vi "SR_Graph_compil_net_param (SubVI).vi"(4 "String":string, 6 "Int32":i32, 7 "String 4":string, 8 "Boolean":bool, 10 "String 2":string, 11 "Boolean 2":bool) -> (3 "String 3":string)   [LabVIEW 2018]
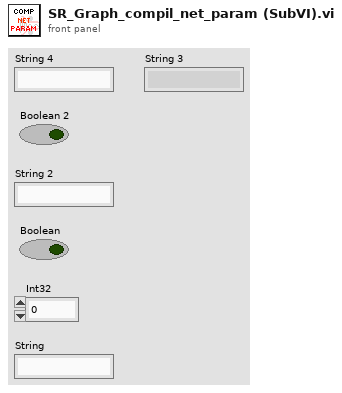
[diagram p1: front panel]
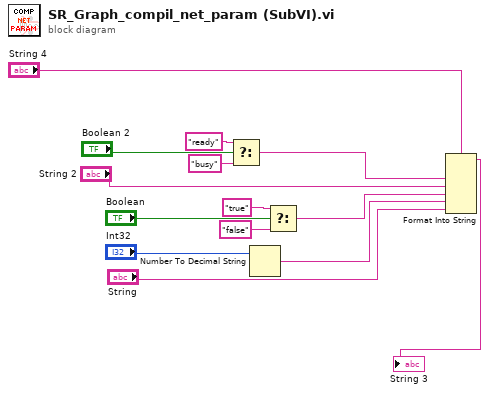
[diagram p0: block diagram]
diagram:
  n1 = Select(t="ready", s="Boolean 2", f="busy") -> (s? t:f=w5:string)
  n2 = Number To Decimal String(number="Int32") -> (decimal integer string=w9:string)  [unwired: 1 in]
  n3 = Select(t="true", s="Boolean", f="false") -> (s? t:f=w8:string)
  n4 = Format Into String(format string="String 4", w5, "String 2", w8, w9, "String") -> (resulting string=→"String 3":string)  [unwired: 2 in, 1 out]
